vi "Control of Pressure.vi"() -> ()   [LabVIEW 2011]
uses:
  Labview/Kelvinox drivers/ITCAPPS.LLB/ITCSetupArray.ctl
  Labview/Kelvinox drivers/ITCAPPS.LLB/ITCSetup.ctl
  Labview/Kelvinox drivers/ITCSUBS.LLB/ITCIO.ctl
  Labview/Kelvinox drivers/BUSGEN.LLB/OxfordAddress.ctl
  Labview/Kelvinox drivers/ITCSUBS.LLB/ITCVersion.ctl
  Global 2.vi
panel:
  out "Percentage":string="7.1953%\r"
  out "Needle valve Open":dbl(slide)=7.1953 scale=0.0..10.0
  in  "Setpoint (mb)":dbl=8.0
  in  "Setpoint":bool
  out "Pressure graph":T1(graph)=[{"Control X axis"=[3632900447.778145, 3632900448.7301993, 3632900449.682254, 3632900450.6533093, 3632900451.6383653, 3632900452.639423, 3632900453.672482, 3632900454.6475377, 3632900455.646595, 3632900456.6726537, 3632900457.673711, 3632900458.651767, 3632900459.6468234, 3632900460.717885, 3632900461.648938, 3632900462.6499953, 3632900463.6510525, 3632900464.6111073, 3632900465.692169, 3632900466.643224, 3632900467.644281, 3632900468.6653395, 3632900469.6763973, 3632900470.667454, 3632900471.6785116, 3632900472.640567, 3632900473.6506243, 3632900474.671683, 3632900475.6227374, 3632900476.683798, 3632900477.6748548, 3632900478.6859126, 3632900479.655968, 3632900480.6570253, 3632900481.6580825, 3632900482.679141, 3632900483.6511965, 3632900484.6612544, 3632900485.692313, 3632900486.643368, 3632900487.6554255, 3632900488.654483, 3632900489.679541, 3632900490.686599, 3632900491.6576543, 3632900492.6747127, 3632900493.6497684, 3632900494.6498256, 3632900495.651883, 3632900496.6789417, 3632900497.642997, 3632900498.644054, 3632900499.655112, 3632900500.6761703], "Control Y axis"=[6.174, 6.161, 6.1513, 6.1301, 6.1114, 6.0978, 6.0764, 6.0557, 6.0374, 6.0213, 5.9999, 5.9733, 5.9517, 5.9344, 5.9177, 5.9149, 5.9215, 5.9347, 5.9468, 5.9494, 5.931, 5.9078, 5.9098, 6.0338, 6.3982, 6.8426, 7.205, 7.4996, 7.8318, 8.2177, 8.54, 8.8112, 9.055, 9.2671, 9.4724, 9.6706, 9.8694, 10.059, 10.2481, 10.4229, 10.5539, 10.6767, 10.755, 10.7956, 10.8063, 10.7869, 10.7381, 10.661, 10.5724, 10.4729, 10.3543, 10.2379, 10.1269, 10.0028]}]
  in  "ITC Setup(write)":T2=[{"Description"="", "IO Info"={"Address"={"Com Port"=1, "ISOBUS Address"=1, "GPIB Address"=0, "Communication"=enum."ISOBUS"}, "Version"=enum."ITC503", "Ch 1 dec places"=0, "Ch 2 dec places"=0, "Ch 3 dec places"=0, "Ch1 Name"="", "Ch2 Name"="", "Ch3 Name"=""}}]
  out "Pressure [mb]":dbl=10.0028
  out "P array":dbl[](array[numeric])=[6.174, 6.161, 6.1513, 6.1301, 6.1114, 6.0978, 6.0764, 6.0557, 6.0374, 6.0213, 5.9999, 5.9733, 5.9517, 5.9344, 5.9177, 5.9149, 5.9215, 5.9347, 5.9468, 5.9494, 5.931, 5.9078, 5.9098, 6.0338, 6.3982, 6.8426, 7.205, 7.4996, 7.8318, 8.2177, 8.54, 8.8112, 9.055, 9.2671, 9.4724, 9.6706, 9.8694, 10.059, 10.2481, 10.4229, 10.5539, 10.6767, 10.755, 10.7956, 10.8063, 10.7869, 10.7381, 10.661, 10.5724, 10.4729, 10.3543, 10.2379, 10.1269, 10.0028]
  in  "Comments":string
  in  "stop":bool
  in  "Delay (min.)":dbl=0.01
  in  "Record":bool
  in  "File Name":path
  out "Time":string="12:01:40"
  out "Time":dbl[](array[numeric])=[3632900447.778145, 3632900448.7301993, 3632900449.682254, 3632900450.6533093, 3632900451.6383653, 3632900452.639423, 3632900453.672482, 3632900454.6475377, 3632900455.646595, 3632900456.6726537, 3632900457.673711, 3632900458.651767, 3632900459.6468234, 3632900460.717885, 3632900461.648938, 3632900462.6499953, 3632900463.6510525, 3632900464.6111073, 3632900465.692169, 3632900466.643224, 3632900467.644281, 3632900468.6653395, 3632900469.6763973, 3632900470.667454, 3632900471.6785116, 3632900472.640567, 3632900473.6506243, 3632900474.671683, 3632900475.6227374, 3632900476.683798, 3632900477.6748548, 3632900478.6859126, 3632900479.655968, 3632900480.6570253, 3632900481.6580825, 3632900482.679141, 3632900483.6511965, 3632900484.6612544, 3632900485.692313, 3632900486.643368, 3632900487.6554255, 3632900488.654483, 3632900489.679541, 3632900490.686599, 3632900491.6576543, 3632900492.6747127, 3632900493.6497684, 3632900494.6498256, 3632900495.651883, 3632900496.6789417, 3632900497.642997, 3632900498.644054, 3632900499.655112, 3632900500.6761703]
  out "REC memory":bool
  # "The pressure setpoint is by default 5mb. We can change this value only directly on ITC"
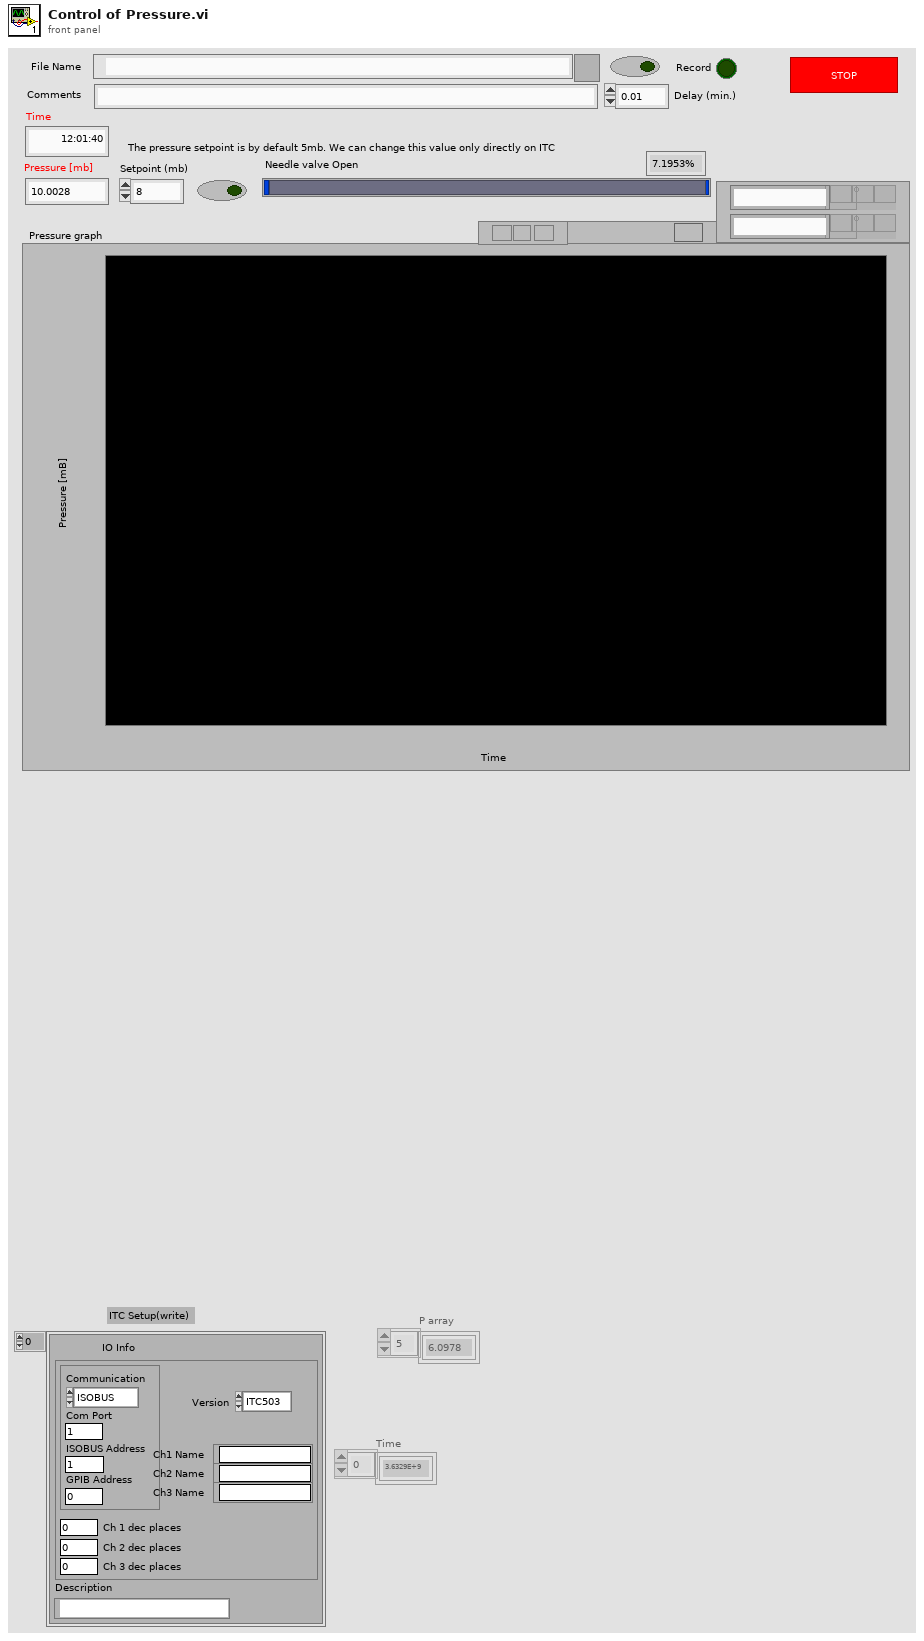
[diagram p1: front panel]
types:
  T1 = cluster{"Control X axis":dbl[], "Control Y axis":dbl[]}[]
  T2 = typedef "ITCSetupArray.ctl" = T3[]
  T3 = typedef "ITCSetup.ctl" = cluster{"Description":string, "IO Info":T4}
  T4 = typedef "ITCIO.ctl" = cluster{"Address":T5, "Version":T6, "Ch 1 dec places":i16, "Ch 2 dec places":i16, "Ch 3 dec places":i16, "Ch1 Name":string, "Ch2 Name":string, "Ch3 Name":string}
  T5 = typedef "OxfordAddress.ctl" = cluster{"Com Port":i32, "ISOBUS Address":i32, "GPIB Address":i16, "Communication":enum16{"RS232", "ISOBUS", "GPIB", "Gateway"}}
  T6 = typedef "ITCVersion.ctl" = enum16{"ITC502", "ITC503", "ITC601"}
  T7 = cluster{"ITC Setup(write)[0]":T3, "ITC Setup(write)[1]":T3, "ITC Setup(write)[2]":T3, "ITC Setup(write)[3]":T3, "ITC Setup(write)[4]":T3, "ITC Setup(write)[5]":T3, "ITC Setup(write)[6]":T3, "ITC Setup(write)[7]":T3, "ITC Setup(write)[8]":T3}
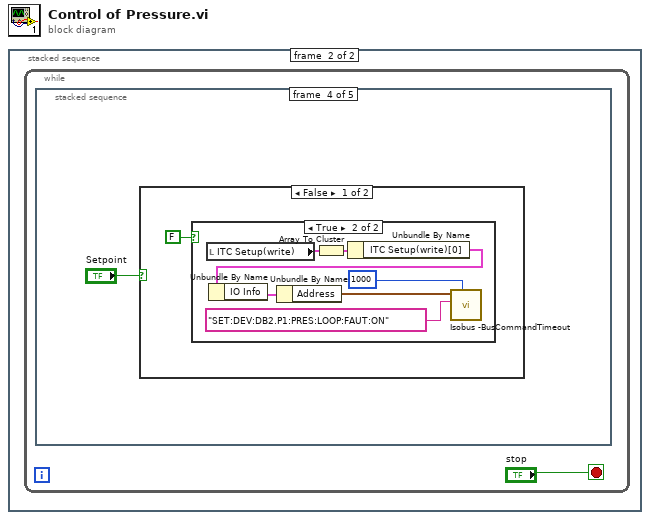
[diagram p0: block diagram]
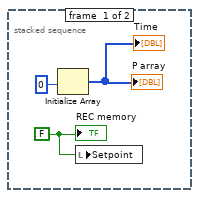
[diagram p2: hidden frame]
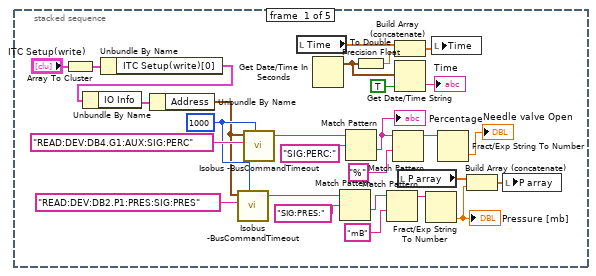
[diagram p3: hidden frame]
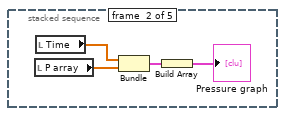
[diagram p4: hidden frame]
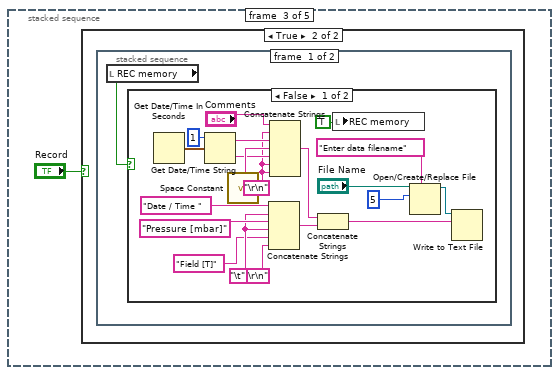
[diagram p5: hidden frame]
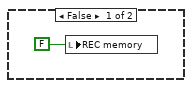
[diagram p6: hidden frame]
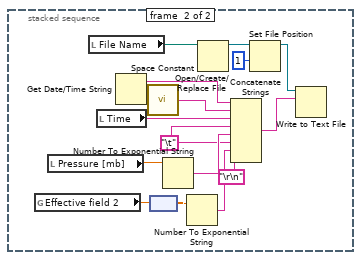
[diagram p8: hidden frame]
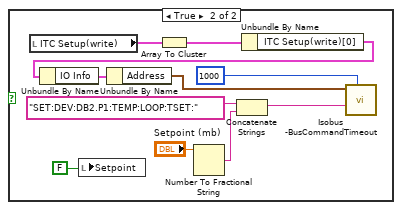
[diagram p10: hidden frame]
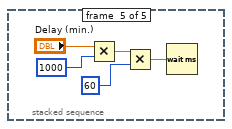
[diagram p11: hidden frame]
diagram:
  n1 = stacked-sequence {
    frame #0 {
      w1 = FALSE
      n2 = Initialize Array(0) -> (→"Time" →"P array":i32[])  [unwired: 1 in]
      n3 = local write "Setpoint"(w1) -> ()
      "REC memory" <- w1
    }
    frame #1 {
      n4 = while {
        stop <- "stop" stop-if-true
        n5 = stacked-sequence {
          frame #0 {
            w9 = u32 1000
            n6 = Array To Cluster(array="ITC Setup(write)") -> (cluster=w23:T7)
            n7 = Unbundle By Name(w23) -> ("ITC Setup(write)[0]"=w21:T3)
            n8 = Unbundle By Name(w21) -> ("IO Info"=w22:T4)
            n9 = Unbundle By Name(w22) -> ("Address"=w8:T5)
            n10 = call "Isobus -BusCommandTimeout.vi"("Timeout (ms)"=w9, "Command"="READ:DEV:DB2.P1:PRES:SIG:PRES", "Address"=w8) -> ("Reply"=w15:string)  [unwired: 5 out]
            n11 = call "Isobus -BusCommandTimeout.vi"("Timeout (ms)"=w9, "Command"="READ:DEV:DB4.G1:AUX:SIG:PERC", "Address"=w8) -> ("Reply"=w10:string)  [unwired: 5 out]
            n12 = local read "Time"() -> (w32:dbl[])
            n13 = Get Date/Time In Seconds() -> (seconds since 1Jan1904=w29:timestamp)
            n14 = Match Pattern(string=w15, regular expression="SIG:PRES:") -> (after substring=w17:string)  [unwired: 1 in, 3 out]
            n15 = Match Pattern(string=w10, regular expression="SIG:PERC:") -> (after substring=w5:string)  [unwired: 1 in, 3 out]
            "Percentage" <- w5
            n16 = To Double Precision Float(number=w29) -> (double precision float=w30:dbl)
            n17 = Match Pattern(string=w17, regular expression="mB") -> (before substring=w19:string)  [unwired: 1 in, 3 out]
            n18 = Match Pattern(string=w5, regular expression="%") -> (before substring=w7:string)  [unwired: 1 in, 3 out]
            n19 = Build Array (concatenate)(w32, w30) -> (w31:dbl[])
            n20 = Get Date/Time String(seconds (now)=w29, want seconds? (F)=TRUE) -> (time string=→"Time":string)  [unwired: 1 in, 1 out]
            n21 = local read "P array"() -> (w25:dbl[])
            n22 = Fract/Exp String To Number(string=w19) -> (number=w14:dbl)  [unwired: 3 in, 1 out]
            "Pressure [mb]" <- w14
            n23 = local write "Time"(w31) -> ()
            n24 = Fract/Exp String To Number(string=w7) -> (number=→"Needle valve Open":dbl)  [unwired: 3 in, 1 out]
            n25 = Build Array (concatenate)(w25, w14) -> (w26:dbl[])
            n26 = local write "P array"(w26) -> ()
          }
          frame #1 {
            n27 = local read "P array"() -> (w35:dbl[])
            n28 = local read "Time"() -> (w36:dbl[])
            n29 = Bundle("Time"=w36, "P array"=w35) -> (w34:cluster{"Time":dbl[], "P array":dbl[]})  [unwired: 1 in]
            n30 = Build Array(w34) -> (→"Pressure graph":cluster{"Time":dbl[], "P array":dbl[]}[])
          }
          frame #2 {
            n31 = case shown="True" "Record" {
              frame False {
                n32 = local write "REC memory"(FALSE) -> ()
              }
              frame True {
                n33 = stacked-sequence {
                  frame #0 {
                    n34 = local read "REC memory"() -> (w39:bool)
                    n35 = case shown="False" w39 {
                      frame False {
                        w45 = "\r\n"
                        w43 = "\t"
                        n36 = Get Date/Time In Seconds() -> (seconds since 1Jan1904=w59:timestamp)
                        n37 = Get Date/Time String(date format (0)=1, seconds (now)=w59) -> (date string=w48:string, time string=w46:string)  [unwired: 1 in]
                        n38 = call <vilib>:"Space Constant.vi"() -> ("String"=w47:string)
                        n39 = Concatenate Strings("Date / Time ", w43, "Pressure [mbar]" ("chaîne"), w43, "Field [T]" ("chaîne"), "\r\n") -> (w56:string)
                        n40 = Concatenate Strings("Comments", w45, w48, w47, w46, w45, w45) -> (w57:string)
                        n41 = Concatenate Strings(w57, w56) -> (w55:string)
                        n42 = local write "REC memory"(TRUE) -> ()
                        n43 = Open/Create/Replace File(file path (use dialog)="File Name", prompt="Enter data filename", operation (0:open)=5) -> (refnum out=w50:refnum<file>)  [unwired: 3 in, 2 out]
                        n44 = Write to Text File(file (use dialog)=w50, text=w55) -> ()  [unwired: 2 in, 3 out]
                      }
                      frame True {
                      }
                    }
                  }
                  frame #1 {
                    w67 = "\t"
                    n45 = global read "Global 2.vi" "Effective field 2"() -> (w64:dbl[unit])
                    n46 = local read "Pressure [mb]"() -> (w65:dbl)
                    n47 = local read "File Name"() -> (w73:path)
                    n48 = local read "Time"() -> (w62:string)
                    n49 = Get Date/Time String() -> (date string=w60:string)  [unwired: 3 in, 1 out]
                    n50 = call <vilib>:"Space Constant.vi"() -> ("String"=w61:string)
                    n51 = node(w64) -> (w63:dbl)
                    n52 = Number To Exponential String(number=w65) -> (E-format string=w69:string)  [unwired: 3 in]
                    n53 = Number To Exponential String(number=w63) -> (E-format string=w66:string)  [unwired: 3 in]
                    n54 = Open/Create/Replace File(file path (use dialog)=w73) -> (refnum out=w72:refnum<file>)  [unwired: 5 in, 2 out]
                    n55 = Concatenate Strings(w60, w61, w62, w67, w69, w67, w66, "\r\n") -> (w74:string)
                    n56 = Set File Position(refnum=w72, from (0:start)=1) -> (refnum out=w71:refnum<file>)  [unwired: 2 in, 1 out]
                    n57 = Write to Text File(file (use dialog)=w71, text=w74) -> ()  [unwired: 2 in, 3 out]
                  }
                }
              }
            }
          }
          frame #3 {
            n58 = case shown="False" "Setpoint" {
              frame False {
                n59 = case shown="True" FALSE {
                  frame False {
                  }
                  frame True {
                    n60 = local read "ITC Setup(write)"() -> (w81:T2)
                    n61 = Array To Cluster(array=w81) -> (cluster=w79:T7)
                    n62 = Unbundle By Name(w79) -> ("ITC Setup(write)[0]"=w80:T3)
                    n63 = Unbundle By Name(w80) -> ("IO Info"=w78:T4)
                    n64 = Unbundle By Name(w78) -> ("Address"=w82:T5)
                    n65 = call "Isobus -BusCommandTimeout.vi"("Timeout (ms)"=u32 1000, "Command"="SET:DEV:DB2.P1:PRES:LOOP:FAUT:ON", "Address"=w82) -> ()  [unwired: 6 out]
                  }
                }
              }
              frame True {
                n66 = local read "ITC Setup(write)"() -> (w93:T2)
                n67 = local write "Setpoint"(FALSE) -> ()
                n68 = Array To Cluster(array=w93) -> (cluster=w90:T7)
                n69 = Number To Fractional String(number="Setpoint (mb)") -> (F-format string=w86:string)  [unwired: 3 in]
                n70 = Concatenate Strings("SET:DEV:DB2.P1:TEMP:LOOP:TSET:", w86) -> (w87:string)
                n71 = Unbundle By Name(w90) -> ("ITC Setup(write)[0]"=w89:T3)
                n72 = Unbundle By Name(w89) -> ("IO Info"=w92:T4)
                n73 = Unbundle By Name(w92) -> ("Address"=w91:T5)
                n74 = call "Isobus -BusCommandTimeout.vi"("Timeout (ms)"=u32 1000, "Command"=w87, "Address"=w91) -> ()  [unwired: 6 out]
              }
            }
          }
          frame #4 {
            n75 = Multiply(x="Delay (min.)", y=1000) -> (x*y=w96:dbl)
            n76 = Multiply(x=w96, y=60) -> (x*y=w95:dbl)
            n77 = Wait (ms)(milliseconds to wait=w95) -> ()  [unwired: 1 out]
          }
        }
      }
    }
  }
